vi "crc.vi"(1 "Input string":string) -> (0 "Output (with crc)":string)   [LabVIEW 2012]
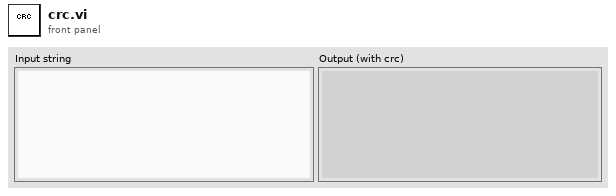
[diagram p1: front panel]
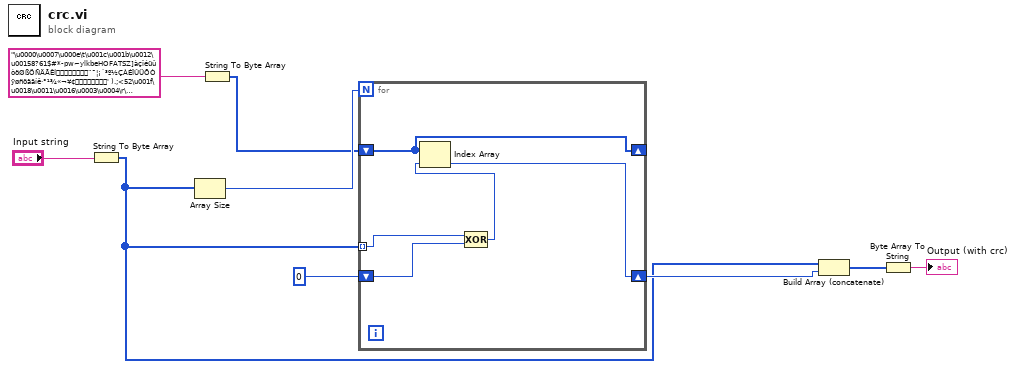
[diagram p0: block diagram]
diagram:
  n1 = String To Byte Array(string="Input string") -> (unsigned byte array=w4:u8[])
  n2 = Array Size(array=w4) -> (size(s)=w6:i32)
  n3 = String To Byte Array(string="\u0000\u0007\u000e\t\u001c\u001b\u0012\u00158?61$#*-pw~ylkbeHOFATSZ]àçîéüûòõØßÖÑÄÃÊÍ¨¯¦¡´³º½ÇÀÉÎÛÜÕÒÿøñöãäíê·°¹¾«¬¥¢' ).;<52\u001f\u0018\u0011\u0016\u0003\u0004\r\nWPY^KLEBohafst}z±¶¿¸­ª£¤ùþ÷ðåâëìÁÆÏÈÝÚÓÔing`ur{|QV_XMJCD\u0019\u001e\u0017\u0010\u0005\u0002\u000b\f!&/(=:34NI@GRU\\[vqxjmdc>907\"%,+\u0006\u0001\b\u000f\u001a\u001d\u0014\u0013®© §²µ¼»ÞÙÐ×ÂÅÌËæáèïúýôó") -> (unsigned byte array=w1:u8[])
  n4 = for {
    N: w6 -> [_]
    shift-right: [w10] -> _
    shift-left: w1 -> [w10]
    shift-right: [w11] -> w5
    shift-left: u8 0 ("element") -> [w13]
    tunnel: w4 -> [w14] mode=indexing
    n5 = Compound Arithmetic op=XOR(w14, w13) -> (w12:u8)
    n6 = Index Array(array=w10, index=w12) -> (element=w11:u8)
  }
  n7 = Build Array (concatenate)(w4, w5) -> (w3:u8[])
  n8 = Byte Array To String(unsigned byte array=w3) -> (string=→"Output (with crc)":string)
